vi "Initalize Runtime Keys.vi"(8 "error in (no error)":errorcluster, 11 "E2E configuration":refnum<class "E2E Tag Exchange configuration.lvclass">) -> (0 "error out":errorcluster, 3 "E2E configuration out":refnum<class "E2E Tag Exchange configuration.lvclass">)   [LabVIEW 2015, in "E2E Tag Exchange configuration.lvclass"]
uses:
  module/configuration/E2E Tag Exchange configuration.lvclass
  module/configuration/E2E Tag Exchange configuration.lvclass/E2E Tag Exchange configuration.ctl
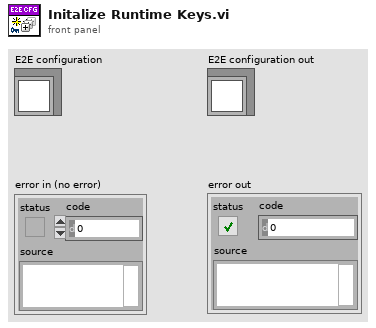
[diagram p1: front panel]
types:
  T1 = typedef "E2E Tag Exchange configuration.lvclass/Runtime Implementation.ctl" = enum16{"RT FIFO", "UDP"}
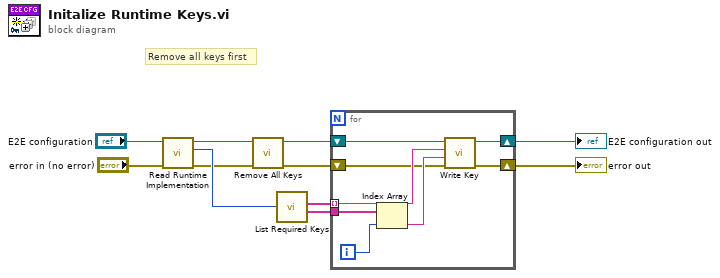
[diagram p0: block diagram]
diagram:
  # "Remove all keys first"
  n1 = call "Read Runtime Implementation.vi"("error in (no error)"="error in (no error)", "E2E Tag Exchange configuration in"="E2E configuration") -> ("error out"=w6:errorcluster, "Runtime Implementation"=w8:T1, "E2E Tag Exchange configuration out"=w7:refnum<class "E2E Tag Exchange configuration.lvclass">)  [unwired: 7 in]
  n2 = call "Remove All Keys.vi"("error in"=w6, "E2E configuration in"=w7) -> ("error out"=w5:errorcluster, "E2E configuration out"=w4:refnum<class "E2E Tag Exchange configuration.lvclass">)  [unwired: 8 in]
  n3 = call "List Required Keys.vi"("Runtime Implementation"=w8) -> ("Initial Values"=w10:string[], "Requested Keys"=w11:string[])  [unwired: 9 in]
  n4 = for {
    tunnel: w11 -> [w16] mode=indexing
    tunnel: w10 -> [w19]
    shift-right: [w12] -> w1
    shift-left: w4 -> [w17]
    shift-right: [w13] -> w3
    shift-left: w5 -> [w14]
    i -> [w18]
    n5 = Index Array(array=w19, index=w18) -> (element=w15:string)
    n6 = call "Write Key.vi"("error in"=w14, "Value"=w15, "Key"=w16, "E2E configuration in"=w17) -> ("error out"=w13:errorcluster, "E2E configuration out"=w12:refnum<class "E2E Tag Exchange configuration.lvclass">)  [unwired: 6 in]
  }
  "error out" <- w3
  "E2E configuration out" <- w1
